vi "Populate Subpanels.vi"(8 "error in (no error)":errorcluster, 9 "View Labels (optional)":string[](array[string]), 10 "Views":refnum<class "Message Enqueuer.lvclass">[](array[class]), 11 "TabbedViewManager In":refnum<class "TabbedViewManager.lvclass">) -> (0 "error out":errorcluster, 3 "TabbedViewManager Out":refnum<class "TabbedViewManager.lvclass">)   [LabVIEW 2015, in "TabbedViewManager.lvlib" / "TabbedViewManager.lvclass"]
uses:
  TabbedViewManager.lvclass
  <vilib>/ActorFramework/Message Enqueuer/Message Enqueuer.lvclass
  TabbedViewManager.lvclass/TabbedViewManager.ctl
  IViewable/IViewable Messages/Insert View Msg/Insert View Msg.lvclass/Insert View Msg.ctl
  <vilib>/ActorFramework/Message Enqueuer/Message Enqueuer.lvclass/Message Enqueuer.ctl
  <vilib>/ActorFramework/Message Enqueuer/Enqueue.vi
  <vilib>/ActorFramework/Message Priority Queue/Priority Enqueue.vi
  IViewManager/IViewManager/IViewManager.lvclass
  IViewable/IViewable Messages/Insert View Msg/Insert View Msg.lvclass
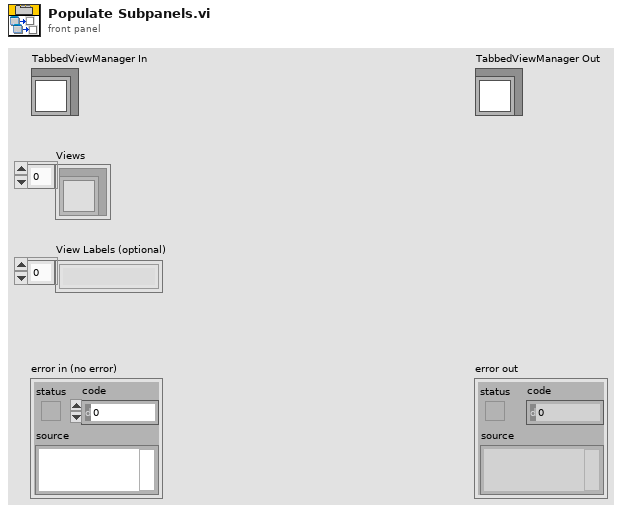
[diagram p1: front panel]
types:
  T1 = enum32{"1", "2", "3", "4", "5", "6", "7", "8", "9", "10"}
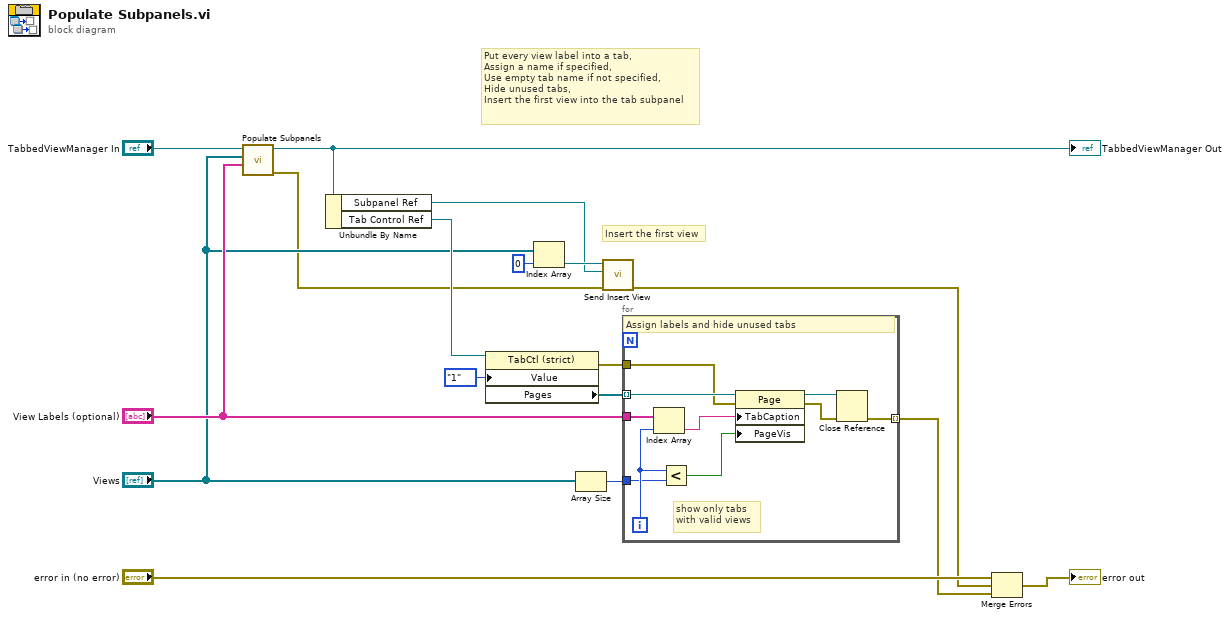
[diagram p0: block diagram]
diagram:
  # "Put every view label into a tab,\nAssign a name if specified,\nUse empty tab name if not specified,\nHide unused tabs,\nInsert the first view into the tab subpanel"
  # "Insert the first view"
  n1 = call-parent "Populate Subpanels.vi"("View Labels (optional)"="View Labels (optional)", "Views"="Views", "IViewManager In"="TabbedViewManager In") -> ("error out"=w4:errorcluster, "IViewManager Out"=w3:refnum<class "TabbedViewManager.lvclass">)  [unwired: 7 in]
  "TabbedViewManager Out" <- w3
  n2 = Unbundle By Name(w3) -> ("Subpanel Ref"=w10:refnum<vi>, "Tab Control Ref"=w11:refnum<vi>)
  n3 = property class="TabCtl (strict)"(reference=w11, "Value"=T1."1") -> (error out=w14:errorcluster, "Pages"=w16:refnum<vi>[])  [unwired: 1 in, 1 out]
  n4 = Index Array(array="Views", index=0) -> (element=w12:refnum<class "Message Enqueuer.lvclass">)
  n5 = Array Size(array="Views") -> (size(s)=w15:i32)
  n6 = call "Send Insert View.vi"("error in (no error)"=w4, "SubPnl Refnum"=w10, "Message Enqueuer"=w12) -> ("error out"=w1:errorcluster)  [unwired: 7 in, 1 out]
  n7 = for {
    tunnel: w16 -> [w27] mode=indexing
    tunnel: "View Labels (optional)" -> [w26]
    tunnel: w15 -> [w23]
    tunnel: w14 -> [w19]
    tunnel: [w18] -> w2 mode=indexing
    i -> [w24]
    # "show only tabs\nwith valid views"
    # "Assign labels and hide unused tabs"
    n8 = Index Array(array=w26, index=w24) -> (element=w25:string)
    n9 = Less?(x=w24, y=w23) -> (x < y?=w22:bool)
    n10 = property class="Page"(reference=w27, error in=w19, "TabCaption"=w25, "PageVis"=w22) -> (reference out=w21:refnum<vi>, error out=w20:errorcluster)
    n11 = Close Reference(reference=w21, error in (no error)=w20) -> (error out=w18:errorcluster)
  }
  n12 = Merge Errors("error in (no error)", w1, w2) -> (→"error out":errorcluster)
